vi "DHE_SaveSyncMacro.vi"(8 "error in":errorcluster) -> (0 "error out":errorcluster)   [LabVIEW 2016]
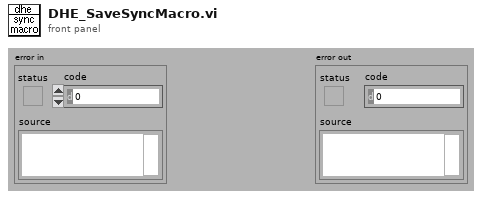
[diagram p1: front panel]
types:
  T1 = typedef "DHE_Img.ctl" = cluster{"title":string, "comment":string, "rootname":string, "imnumber":i32, "mext":bool, "imdir":string, "basename":string, "imprefix":string, "imsufix":string, "froot":string}
  T2 = typedef "DHE_Obs.ctl" = cluster{"observer":string, "obstype":string, "exptime":dbl, "coadds":i32, "fowler":i32, "nimages":i32, "display":bool, "autowrite":bool, "frames to write":cluster{"subs":bool, "reset":bool, "exposed":bool}, "frames to display":cluster{"subs":bool, "reset":bool, "exposed":bool}, "sur":i32}
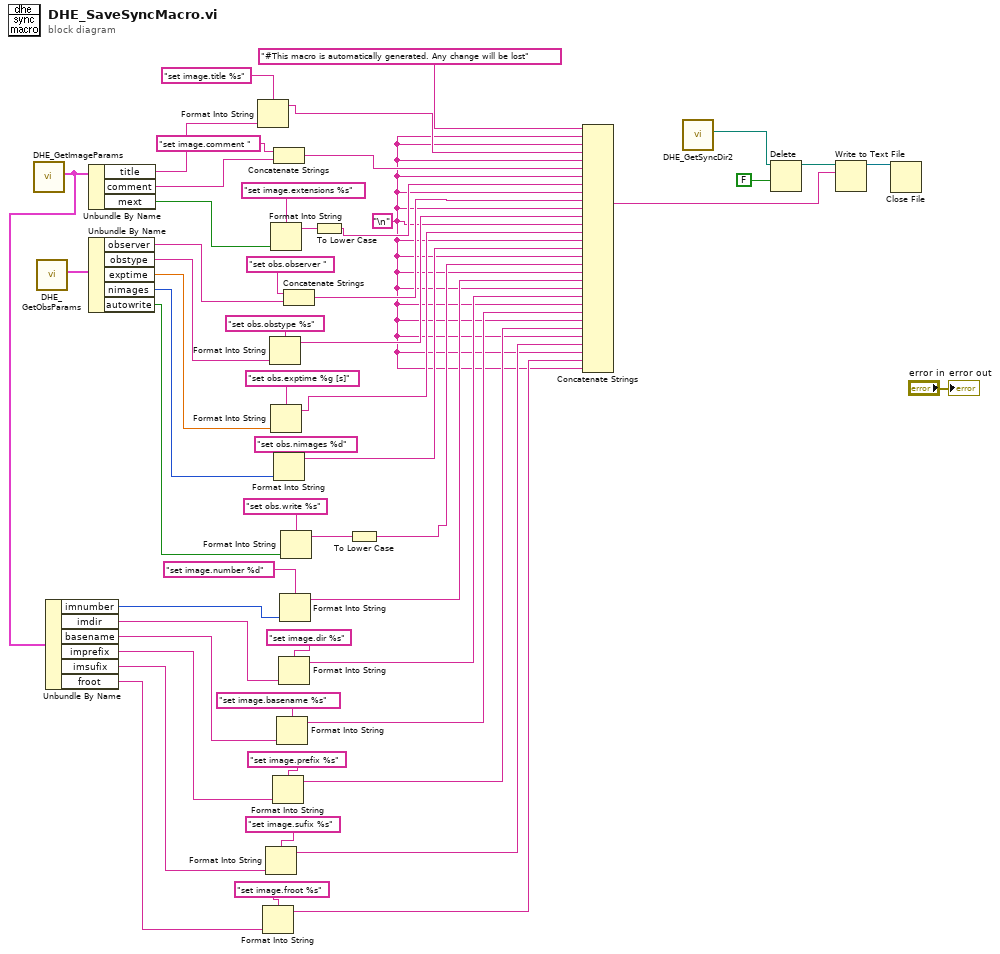
[diagram p0: block diagram]
diagram:
  w2 = "\n"
  n1 = call "DHE_GetImageParams.vi"() -> ("DHE_IMAGE"=w21:T1)  [unwired: 11 out]
  n2 = call "DHE_GetObsParams.vi"() -> ("DHE_OBS"=w54:T2)  [unwired: 11 out]
  n3 = Unbundle By Name(w21) -> ("imnumber"=w19:i32, "imdir"=w17:string, "basename"=w15:string, "imprefix"=w13:string, "imsufix"=w12:string, "froot"=w9:string)
  n4 = Unbundle By Name(w21) -> ("title"=w52:string, "comment"=w50:string, "mext"=w48:bool)
  n5 = Unbundle By Name(w54) -> ("observer"=w46:string, "obstype"=w44:string, "exptime"=w42:dbl, "nimages"=w40:i32, "autowrite"=w38:bool)
  n6 = Format Into String(format string="set image.title %s", w52) -> (resulting string=w37:string)  [unwired: 2 in, 1 out]
  n7 = Format Into String(format string="set image.froot %s", w9) -> (resulting string=w3:string)  [unwired: 2 in, 1 out]
  n8 = Format Into String(format string="set image.sufix %s", w12) -> (resulting string=w4:string)  [unwired: 2 in, 1 out]
  n9 = Format Into String(format string="set obs.obstype %s", w44) -> (resulting string=w33:string)  [unwired: 2 in, 1 out]
  n10 = Format Into String(format string="set image.extensions %s", w48) -> (resulting string=w35:string)  [unwired: 2 in, 1 out]
  n11 = Format Into String(format string="set obs.exptime %g [s]", w42) -> (resulting string=w32:string)  [unwired: 2 in, 1 out]
  n12 = Format Into String(format string="set image.prefix %s", w13) -> (resulting string=w5:string)  [unwired: 2 in, 1 out]
  n13 = Concatenate Strings("set image.comment " ("format string"), w50) -> (w36:string)
  n14 = Format Into String(format string="set obs.nimages %d", w40) -> (resulting string=w31:string)  [unwired: 2 in, 1 out]
  n15 = Format Into String(format string="set image.basename %s", w15) -> (resulting string=w6:string)  [unwired: 2 in, 1 out]
  n16 = Format Into String(format string="set image.dir %s", w17) -> (resulting string=w7:string)  [unwired: 2 in, 1 out]
  n17 = Format Into String(format string="set image.number %d", w19) -> (resulting string=w8:string)  [unwired: 2 in, 1 out]
  n18 = Format Into String(format string="set obs.write %s", w38) -> (resulting string=w30:string)  [unwired: 2 in, 1 out]
  n19 = Concatenate Strings("set obs.observer " ("format string"), w46) -> (w34:string)
  n20 = To Lower Case(string=w35) -> (all lower case string=w22:string)
  n21 = To Lower Case(string=w30) -> (all lower case string=w23:string)
  n22 = Concatenate Strings("#This macro is automatically generated. Any change will be lost" ("string"), w2, w2, w37, w2, w36, w2, w22, w2, w34, w2, w33, w2, w32, w2, w31, w2, w23, w2, w8, w2, w7, w2, w6, w2, w5, w2, w4, w2, w3, w2) -> (w26:string)
  n23 = call "DHE_GetSyncDir2.vi"() -> ("sync file"=w1:path)  [unwired: 11 out]
  n24 = Delete(path (use dialog)=w1, confirm (F)=FALSE) -> (deleted path=w27:path)  [unwired: 1 in, 4 out]
  n25 = Write to Text File(file (use dialog)=w27, text=w26) -> (refnum out=w25:refnum<file>)  [unwired: 1 in, 3 out]
  n26 = Close File(refnum=w25) -> ()  [unwired: 1 in, 2 out]
  "error out" <- "error in"
